vi "GUI Enable Disable.vi"(0 "Connection Ststus":bool, 5 "Search Type":string, 7 "First Run":bool, 9 "Reference":T1, 11 "error in (no error)":errorcluster) -> (15 "error out":errorcluster)   [LabVIEW 2017]
uses:
  Controls/GUI Reference Cluster.ctl
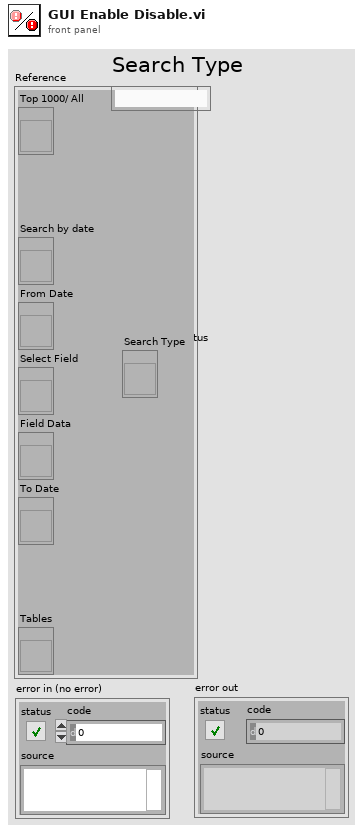
[diagram p1: front panel]
types:
  T1 = typedef "GUI Reference Cluster.ctl" = cluster{"Top 1000/ All":refnum<vi>, "Search by date":refnum<vi>, "From Date":refnum<vi>, "Select Field":refnum<vi>, "Field Data":refnum<vi>, "To Date":refnum<vi>, "Tables":refnum<vi>, "Search Type":refnum<vi>}
  T2 = enum8{"Enabled", "Disabled", "Disabled and Grayed Out"}
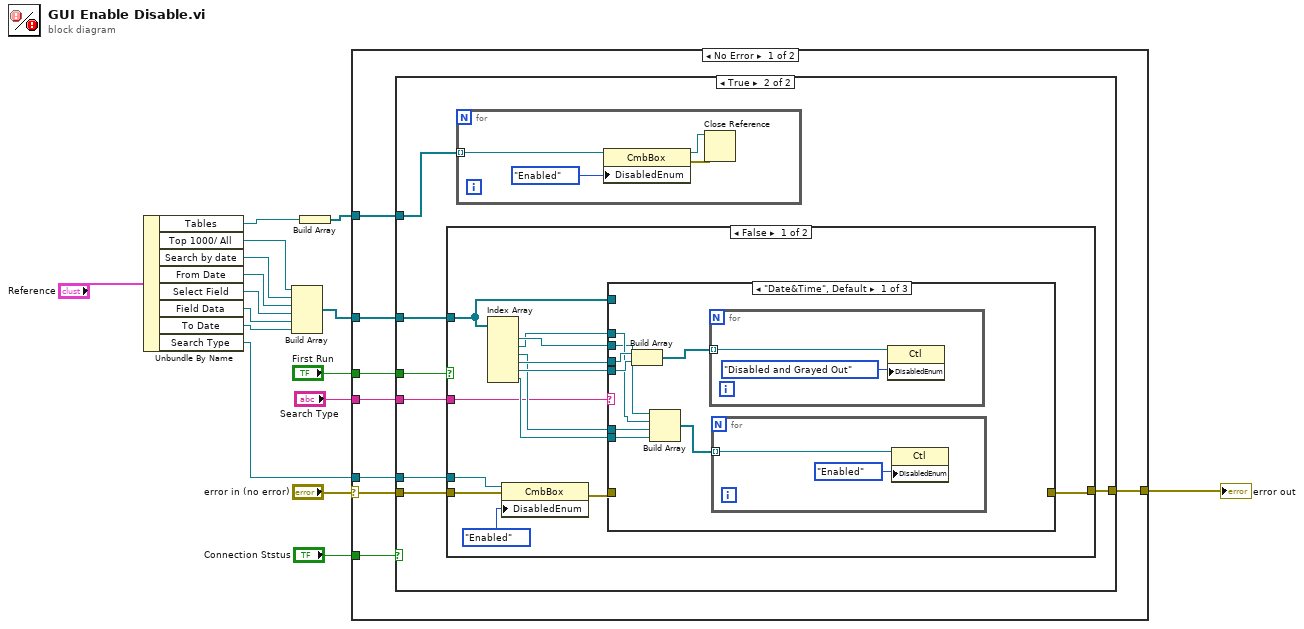
[diagram p0: block diagram]
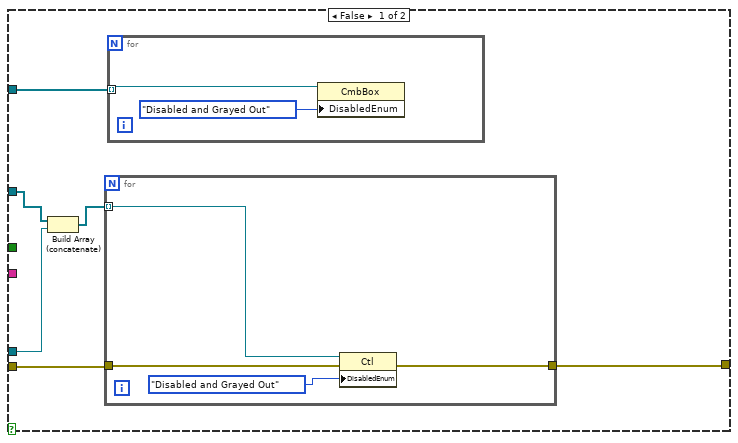
[diagram p2: hidden frame]
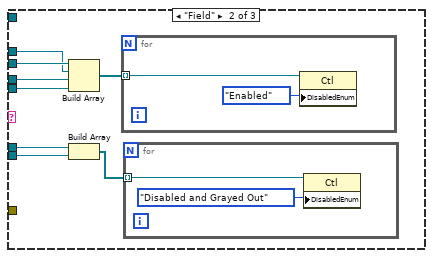
[diagram p3: hidden frame]
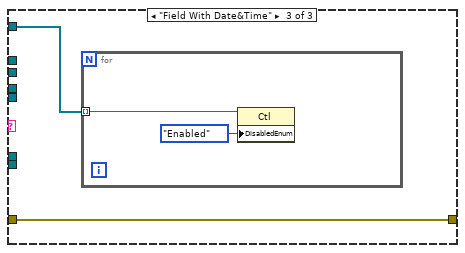
[diagram p4: hidden frame]
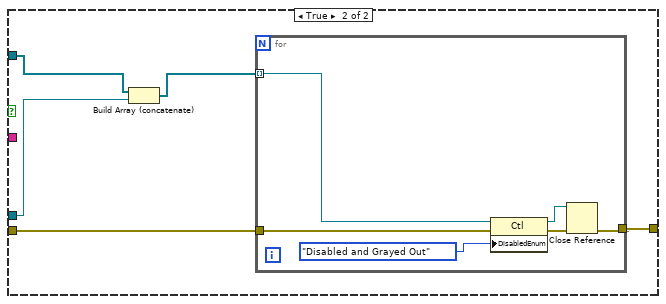
[diagram p5: hidden frame]
diagram:
  n1 = Unbundle By Name("Reference") -> ("Tables"=w4:refnum<vi>, "Top 1000/ All"=w13:refnum<vi>, "Search by date"=w12:refnum<vi>, "From Date"=w11:refnum<vi>, "Select Field"=w10:refnum<vi>, "Field Data"=w9:refnum<vi>, "To Date"=w8:refnum<vi>, "Search Type"=w1:refnum<vi>)
  n2 = Build Array(w13, w12, w11, w10, w9, w8) -> (w7:refnum<vi>[])
  n3 = Build Array(w4) -> (w3:refnum<vi>[])
  n4 = case shown="No Error" "error in (no error)" {
    selector: "error in (no error)" -> [w22 w100]
    tunnel: "First Run" -> [w24 _]
    tunnel: w7 -> [w23 _]
    tunnel: [w21 w100] -> w14
    tunnel: "Connection Ststus" -> [w20 _]
    tunnel: w3 -> [w19 _]
    tunnel: "Search Type" -> [w18 _]
    tunnel: w1 -> [w17 _]
    frame No Error {
      n5 = case shown="True" w20 {
        tunnel: w24 -> [_ w43]
        tunnel: w23 -> [w27 w42]
        tunnel: w22 -> [w29 w41]
        tunnel: [w28 w40] -> w21
        tunnel: w19 -> [w30 w39]
        tunnel: w18 -> [_ w38]
        tunnel: w17 -> [w26 w37]
        frame False {
          n6 = Build Array (concatenate)(w27, w26) -> (w25:refnum<vi>[])
          n7 = for {
            tunnel: w25 -> [w34] mode=indexing
            tunnel: w29 -> [w32]
            tunnel: [w33] -> w28
            n8 = property class="Ctl"(reference=w34, error in=w32, "DisabledEnum"=T2."Disabled and Grayed Out" ("Disabled")) -> (error out=w33:errorcluster)  [unwired: 1 out]
          }
          n9 = for {
            tunnel: w30 -> [w35] mode=indexing
            n10 = property class="CmbBox"(reference=w35, "DisabledEnum"=T2."Disabled and Grayed Out" ("Disabled")) -> ()  [unwired: 1 in, 2 out]
          }
        }
        frame True {
          n11 = case shown="False" w43 {
            tunnel: w42 -> [w55 w91]
            tunnel: w41 -> [w52 w93]
            tunnel: [w54 w92] -> w40
            tunnel: w38 -> [w53 _]
            tunnel: w37 -> [w50 w90]
            frame False {
              n12 = Index Array(array=w55) -> (element #1=w60:refnum<vi>, element #2=w48:refnum<vi>, element #3=w57:refnum<vi>, element #4=w59:refnum<vi>, element #5=w58:refnum<vi>, element #6=w56:refnum<vi>)  [unwired: 6 in]
              n13 = property class="CmbBox"(reference=w50, error in=w52, "DisabledEnum"=T2."Enabled" ("Disabled")) -> (error out=w51:errorcluster)  [unwired: 1 out]
              n14 = case shown="\"Date&Time\", Default" w53 {
                tunnel: w60 -> [w61 w74 _]
                tunnel: w59 -> [w68 w78 _]
                tunnel: w58 -> [w67 w77 _]
                tunnel: w57 -> [w66 w76 _]
                tunnel: w56 -> [w65 w75 _]
                tunnel: w51 -> [_ _ w85]
                tunnel: w55 -> [_ _ w86]
                tunnel: [_ _ w85] -> w54
                tunnel: w48 -> [w62 w73 _]
                frame "Date&Time", Default {
                  n15 = Build Array(w68, w67) -> (w64:refnum<vi>[])
                  n16 = Build Array(w61, w62, w66, w65) -> (w63:refnum<vi>[])
                  n17 = for {
                    tunnel: w64 -> [w72] mode=indexing
                    n18 = property class="Ctl"(reference=w72, "DisabledEnum"=T2."Disabled and Grayed Out" ("Disabled")) -> ()  [unwired: 1 in, 2 out]
                  }
                  n19 = for {
                    tunnel: w63 -> [w69] mode=indexing
                    n20 = property class="Ctl"(reference=w69, "DisabledEnum"=T2."Enabled" ("Disabled")) -> ()  [unwired: 1 in, 2 out]
                  }
                }
                frame "Field" {
                  n21 = Build Array(w74, w73, w78, w77) -> (w80:refnum<vi>[])
                  n22 = Build Array(w76, w75) -> (w79:refnum<vi>[])
                  n23 = for {
                    tunnel: w80 -> [w84] mode=indexing
                    n24 = property class="Ctl"(reference=w84, "DisabledEnum"=T2."Enabled" ("Disabled")) -> ()  [unwired: 1 in, 2 out]
                  }
                  n25 = for {
                    tunnel: w79 -> [w81] mode=indexing
                    n26 = property class="Ctl"(reference=w81, "DisabledEnum"=T2."Disabled and Grayed Out" ("Disabled")) -> ()  [unwired: 1 in, 2 out]
                  }
                }
                frame "Field With Date&Time" {
                  n27 = for {
                    tunnel: w86 -> [w88] mode=indexing
                    n28 = property class="Ctl"(reference=w88, "DisabledEnum"=T2."Enabled" ("Disabled")) -> ()  [unwired: 1 in, 2 out]
                  }
                }
              }
            }
            frame True {
              n29 = Build Array (concatenate)(w91, w90) -> (w89:refnum<vi>[])
              n30 = for {
                tunnel: w89 -> [w99] mode=indexing
                tunnel: w93 -> [w98]
                tunnel: [w94] -> w92
                n31 = property class="Ctl"(reference=w99, error in=w98, "DisabledEnum"=T2."Disabled and Grayed Out" ("Disabled")) -> (reference out=w95:refnum<vi>, error out=w96:errorcluster)
                n32 = Close Reference(reference=w95, error in (no error)=w96) -> (error out=w94:errorcluster)
              }
            }
          }
          n33 = for {
            tunnel: w39 -> [w46] mode=indexing
            n34 = property class="CmbBox"(reference=w46, "DisabledEnum"=T2."Enabled" ("Disabled")) -> (reference out=w44:refnum<vi>, error out=w45:errorcluster)  [unwired: 1 in]
            n35 = Close Reference(reference=w44, error in (no error)=w45) -> ()  [unwired: 1 out]
          }
        }
      }
    }
    frame Error {
    }
  }
  "error out" <- w14
